vi "Xml_Save_Current.vi"(8 "error in (no error)":errorcluster, 11 "Variant":variant) -> (0 "error out":errorcluster)   [LabVIEW 2015]
uses:
  controls/QMH_UI_Cluster.ctl
  controls/QMH_UI_References.ctl
  controls/QMH_UI_Report.ctl
  controls/QMH_UI_Command.ctl
  controls/QMH_ICR_Command.ctl
  controls/QMH_Status.ctl
  controls/EXPERT_Inputs.ctl
  controls/SOFTWARE_Inputs.ctl
  controls/AO_6711_Inputs.ctl
  controls/AWG_5421_Inputs.ctl
  controls/DIGIT_5122_Inputs.ctl
  <instrlib>/niScope/Controls/niScope trigger source.ctl
  controls/HSDIO_6541_Inputs.ctl
  <instrlib>/niHSDIO/niHSDIO.llb/niHSDIO_ctl Trigger Source Values (Ring).ctl
  <vilib>/NI/GXML/GXML.lvlib
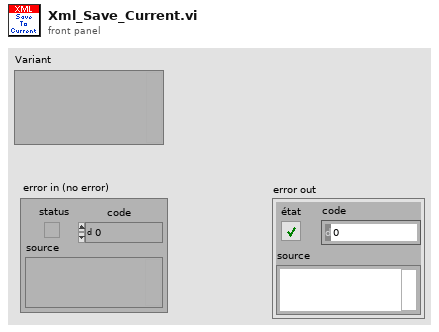
[diagram p1: front panel]
types:
  T1 = typedef "EXPERT_Inputs.ctl" = cluster{"SOFTWARE Inputs":T2, "AO 6711 Inputs":T3, "AWG 5421 Inputs":T4, "DIGIT 5122 Inputs":T5, "HSDIO 6541 Inputs":T7}
  T2 = typedef "SOFTWARE_Inputs.ctl" = cluster{"Application Directory":path, "Resources Path":path, "Data Path":path, "XML Path":path, "XML File Filter":string, "Excit Scripts Path":path, "Excit Scripts File Filter":string, "Excit Waveforms Path":path, "Excit Waveforms File Filter":string, "Timing Scripts Path":path, "Timing Scripts File Filter":string, "Timing Waveforms Path":path, "Timing Waveforms File Filter":string, "Trapping Waveforms Path":path, "Trapping Waveforms File Filter":string}
  T3 = typedef "AO_6711_Inputs.ctl" = cluster{"Physical Channels":tag, "Min Voltage":dbl, "Max Voltage":dbl, "Trigger Source":tag, "counter":tag}
  T4 = typedef "AWG_5421_Inputs.ctl" = cluster{"Resource Name":refnum<k15>, "Trigger Type":u16, "Trigger Source":string, "Sample Rate":dbl}
  T5 = typedef "DIGIT_5122_Inputs.ctl" = cluster{"Sample Rate":dbl, "Resource Name":refnum<k15>, "Channel Name":string, "Trigger Source":T6, "Vertical Range":dbl, "Trigger Level":dbl}
  T6 = typedef "niScope trigger source.ctl" = string
  T7 = typedef "HSDIO_6541_Inputs.ctl" = cluster{"Resource Name":refnum<k15>, "Clock Rate":dbl, "Trigger Source":T8}
  T8 = typedef "niHSDIO_ctl Trigger Source Values (Ring).ctl" = string
  T9 = typedef "QMH_UI_Cluster.ctl" = cluster{"QMH UI References":T10, "QMH UI Report":T11}
  T10 = typedef "QMH_UI_References.ctl" = cluster{"Refnum Load":refnum<vi>, "Refnum Save":refnum<vi>, "Refnum Start":refnum<vi>, "Refnum Stop":refnum<vi>, "Refnum Exit":refnum<vi>, "Refnum Tabs":refnum<vi>, "Refnum SPECTRUM":refnum<vi>, "Refnum EXPERIMENT":refnum<vi>, "Refnum VOLTAGES":refnum<vi>, "Refnum SEQUENCE":refnum<vi>, "Refnum EXPERT":refnum<vi>, "Refnum CHANGE Experiment":refnum<vi>, "Refnum CHANGE Voltages":refnum<vi>, "Refnum CHANGE Sequence":refnum<vi>, "Refnum CHANGE Expert":refnum<vi>}
  T11 = typedef "QMH_UI_Report.ctl" = cluster{"UI Status":T12, "QLA Status":string, "ICR Status":T13, "QMH Status":T14}
  T12 = typedef "QMH_UI_Command.ctl" = enum16{"Initialize", "UI Load", "UI Save", "UI Change Experiment", "UI Change Voltages", "UI Change Sequence", "UI Change Expert", "Ready to Start", "UI Start", "UI Stop", "UI Exit", "Update Report", "Update ICR Report"}
  T13 = typedef "QMH_ICR_Command.ctl" = enum16{"Initialize", "Hardware Setup", "Waiting for Trigger", "Sequence Started", "Sequence Finished", "Writing Data", "Hardware Reset", "Exit"}
  T14 = typedef "QMH_Status.ctl" = enum16{"Init", "Loading", "Setup", "Ready to Start", "Started", "Idle"}
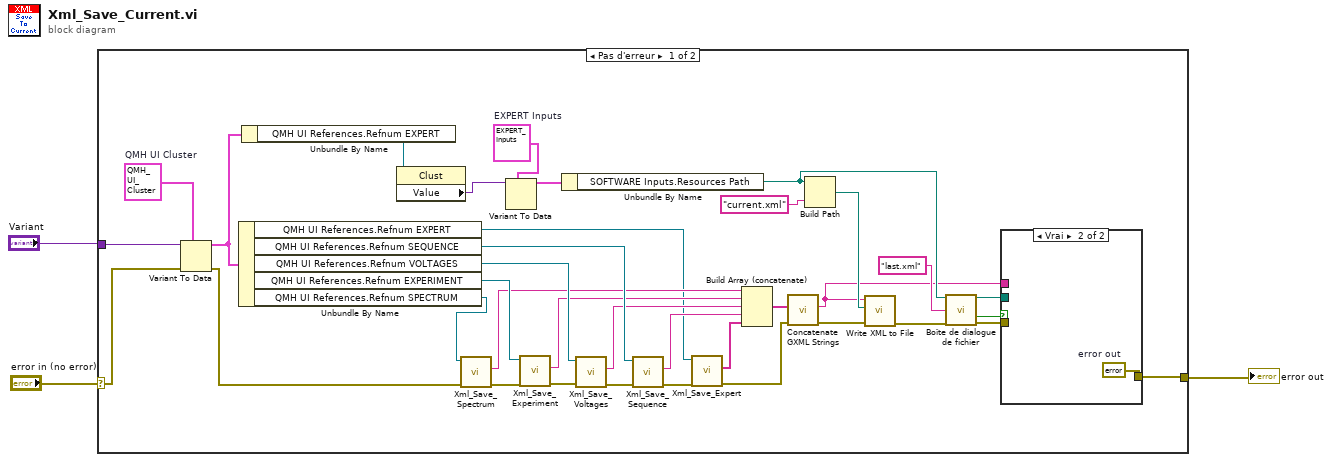
[diagram p0: block diagram]
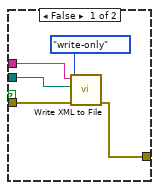
[diagram p2: hidden frame]
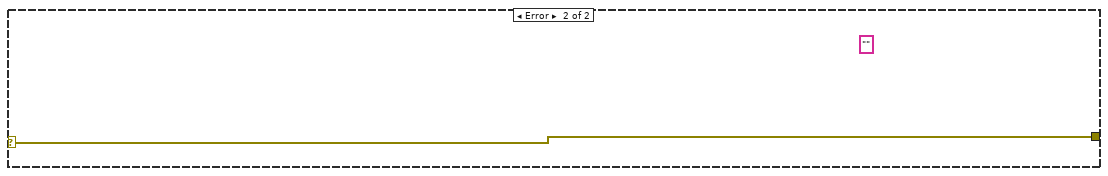
[diagram p3: hidden frame]
diagram:
  n1 = case shown="Pas d'erreur" "error in (no error)" {
    selector: "error in (no error)" -> [w17 w46]
    tunnel: "Variant" -> [w19 _]
    tunnel: [w10 w46] -> w2
    frame No Error {
      w13 = T1 {"SOFTWARE Inputs"={"Application Directory"=path "D:/S.O.F.T.S/LABVIEW/PIL", "Resources Path"=path "D:/S.O.F.T.S/LABVIEW/PIL/resources", "Data Path"=path "D:/PIRENEA/DATA", "XML Path"=path "D:/PIRENEA/DATA", "XML File Filter"="*.xml", "Excit Scripts Path"=path "D:/PIRENEA/EXCIT_SCRIPTS", "Excit Scripts File Filter"="*.txt", "Excit Waveforms Path"=path "D:/PIRENEA/EXCIT_WFMS", "Excit Waveforms File Filter"="*.bin", "Timing Scripts Path"=path "D:/PIRENEA/SEQUENCE_SCRIPTS", "Timing Scripts File Filter"="*.txt", "Timing Waveforms Path"=path "D:/PIRENEA/SEQUENCE_WFMS", "Timing Waveforms File Filter"="*.bin", "Trapping Waveforms Path"=path "D:/PIRENEA/TRAPPING_WFMS", "Trapping Waveforms File Filter"="*.bin"}, "AO 6711 Inputs"={"Physical Channels"="AnalogOutput/ao0:3", "Min Voltage"=-10.0, "Max Voltage"=10.0, "Trigger Source"="/AnalogOutput/PFI0", "counter"="AnalogOutput/ctr0"}, "AWG 5421 Inputs"={"Resource Name"="WaveformGenerator", "Trigger Type"=2, "Trigger Source"="PFI0", "Sample Rate"=20000000.0}, "DIGIT 5122 Inputs"={"Sample Rate"=10000000.0, "Resource Name"="Digitizer", "Channel Name"="0", "Trigger Source"="VAL_EXTERNAL", "Vertical Range"=10.0, "Trigger Level"=3.0}, "HSDIO 6541 Inputs"={"Resource Name"="SequencerHSDIO", "Clock Rate"=1000000.0, "Trigger Source"="PFI0"}}  # EXPERT Inputs
      w18 = T9 {"QMH UI References"={"Refnum Load"=refnum, "Refnum Save"=refnum, "Refnum Start"=refnum, "Refnum Stop"=refnum, "Refnum Exit"=refnum, "Refnum Tabs"=refnum, "Refnum SPECTRUM"=refnum, "Refnum EXPERIMENT"=refnum, "Refnum VOLTAGES"=refnum, "Refnum SEQUENCE"=refnum, "Refnum EXPERT"=refnum, "Refnum CHANGE Experiment"=refnum, "Refnum CHANGE Voltages"=refnum, "Refnum CHANGE Sequence"=refnum, "Refnum CHANGE Expert"=refnum}, "QMH UI Report"={"UI Status"=enum."Initialize", "QLA Status"="", "ICR Status"=enum."Initialize", "QMH Status"=enum."Init"}}  # QMH UI Cluster
      n2 = Variant To Data(error in=w17, type=w18, Variant=w19) -> (data=w16:T9, error out=w4:errorcluster)
      n3 = Unbundle By Name(w16) -> ("QMH UI References.Refnum EXPERT"=w20:refnum<vi>, "QMH UI References.Refnum SEQUENCE"=w37:refnum<vi>, "QMH UI References.Refnum VOLTAGES"=w38:refnum<vi>, "QMH UI References.Refnum EXPERIMENT"=w39:refnum<vi>, "QMH UI References.Refnum SPECTRUM"=w26:refnum<vi>)
      n4 = Unbundle By Name(w16) -> ("QMH UI References.Refnum EXPERT"=w15:refnum<vi>)
      n5 = property class="Clust"(reference=w15) -> ("Value"=w14:variant)  [unwired: 1 in, 2 out]
      n6 = call "Xml_Save_Spectrum.vi"("error in (no error)"=w4, "Refnum Clust"=w26) -> ("error out"=w28:errorcluster, "XML String Out"=w27:string)  [unwired: 8 in]
      n7 = Variant To Data(type=w13, Variant=w14) -> (data=w12:T1)  [unwired: 1 in, 1 out]
      n8 = call "Xml_Save_Experiment.vi"("error in (no error)"=w28, "Refnum Clust"=w39) -> ("error out"=w25:errorcluster, "XML String Out"=w33:string)  [unwired: 8 in]
      n9 = Unbundle By Name(w12) -> ("SOFTWARE Inputs.Resources Path"=w8:path)
      n10 = call "Xml_Save_Voltages.vi"("error in (no error)"=w25, "Refnum Clust"=w38) -> ("error out"=w24:errorcluster, "XML String Out"=w34:string)  [unwired: 8 in]
      n11 = call "Xml_Save_Sequence.vi"("error in (no error)"=w24, "Refnum Clust"=w37) -> ("error out"=w23:errorcluster, "XML String Out"=w35:string)  [unwired: 8 in]
      n12 = call "Xml_Save_Expert.vi"("error in (no error)"=w23, "Refnum Clust"=w20) -> ("error out"=w31:errorcluster, "XML String Out"=w36:string[])  [unwired: 8 in]
      n13 = Build Array (concatenate)(w27, w33, w34, w35, w36) -> (w32:string[])
      n14 = call <vilib>:"Concatenate GXML Strings.vi"("error in"=w31, "GXML Strings"=w32) -> ("error out"=w9:errorcluster, "Concatenated GXML String"=w6:string)  [unwired: 8 in]
      n15 = Build Path(base path=w8, name or relative path="current.xml" ("nom ou chemin relatif")) -> (appended path=w7:path)
      n16 = call <vilib>:"Write XML to File.vi"("error in"=w9, "XML File Path"=w7, "XML Input"=w6) -> ("error out"=w5:errorcluster)  [unwired: 8 in]
      n17 = call "Boîte de dialogue de fichier"("start path"=w8, "default name"="last.xml", "error in"=w5) -> ("selected path"=w29:path, "cancelled"=w22:bool, "error out"=w30:errorcluster)  [unwired: 9 in, 1 out]
      n18 = case shown="Vrai" w22 {
        tunnel: w30 -> [w44 _]
        tunnel: w6 -> [w43 _]
        tunnel: w29 -> [w42 _]
        tunnel: [w40 w45] -> w10
        frame False {
          n19 = call <vilib>:"Write XML to File.vi"("error in"=w44, "file access"=enum16{"read/write", "read-only", "write-only"}."write-only", "XML File Path"=w42, "XML Input"=w43) -> ("error out"=w40:errorcluster)  [unwired: 7 in]
        }
        frame True {
          w45 = errorcluster {"status"=FALSE, "code"=0, "source"=""}  # error out
        }
      }
    }
    frame Error {
      (unwired) "" ("XML String Out")
    }
  }
  "error out" <- w2
